vi "LibraryTest.vi"() -> ()   [LabVIEW 2019]
uses:
  <vilib>/ptbypt/NI_PtbyPt.lvlib
panel:
  in  "ipAddress 2":string="192.168.254.1"
  out "Sample dt (ms)":dbl format="%0.2f"
  in  "stop":bool
  out "length":i32
  out "error out":errorcluster
  out "return 2":string
  out "qtmPort":i32
  out "ipAddress":string
  out "return":i32
  # "IP Address of the PC running QTM"
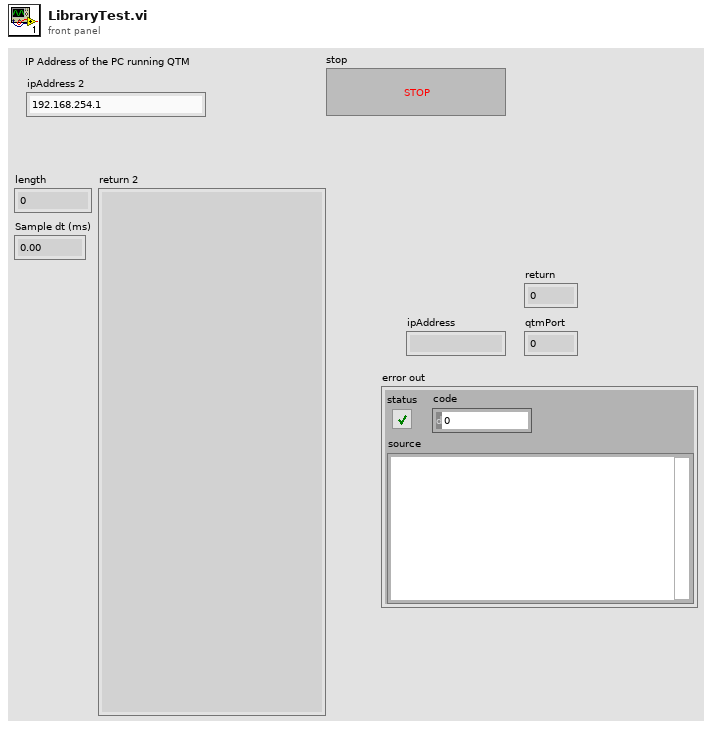
[diagram p1: front panel]
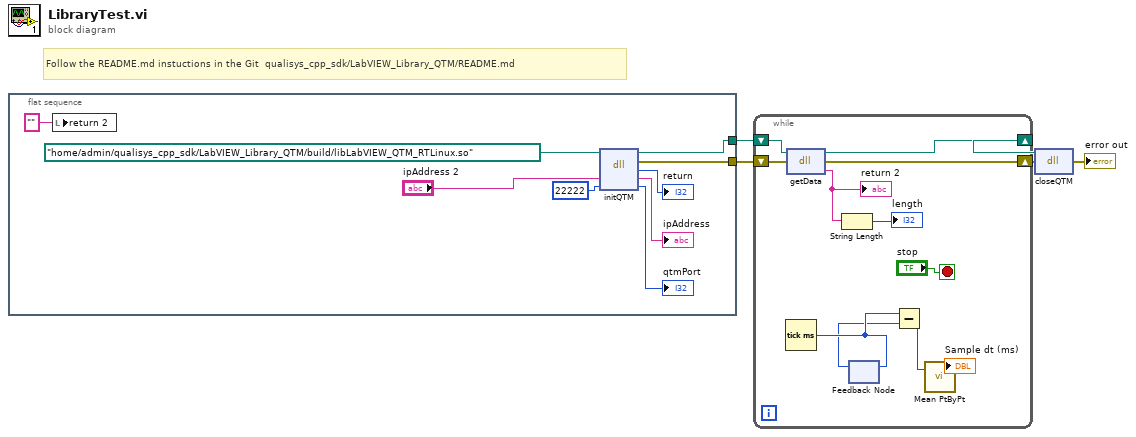
[diagram p0: block diagram]
diagram:
  # "Follow the README.md instuctions in the Git  qualisys_cpp_sdk/LabVIEW_Library_QTM/README.md"
  n1 = flat-sequence {
    tunnel: [w8] -> w5
    tunnel: [w7] -> w3
    frame #0 {
      n2 = local write "return 2"("") -> ()
      n3 = dll-call lib="home/admin/qualisys_cpp_sdk/LabVIEW_Library_QTM/build/libLabVIEW_QTM_RTLinux.so" fn="initQTM"(path in=path "/home/admin/qualisys_cpp_sdk/LabVIEW_Library_QTM/build/libLabVIEW_QTM_RTLinux.so", "ipAddress"="ipAddress 2", "qtmPort"=22222) -> (path out=w8:path, error out=w7:errorcluster, "return"=→"return":i32, "ipAddress"=→"ipAddress":string, "qtmPort"=→"qtmPort":i32)  [unwired: 2 in]
    }
  }
  n4 = while {
    shift-right: [w24] -> w4
    shift-left: w5 -> [w25]
    shift-right: [w22] -> w2
    shift-left: w3 -> [w23]
    stop <- "stop" stop-if-true
    n5 = Tick Count (ms)() -> (millisecond timer value=w18:u32)
    n6 = dll-call lib="home/admin/qualisys_cpp_sdk/LabVIEW_Library_QTM/build/libLabVIEW_QTM_RTLinux.so" fn="getData"(path in=w25, error in=w23) -> (path out=w24:path, error out=w22:errorcluster, "return"=w20:string)  [unwired: 1 in]
    "return 2" <- w20
    n7 = String Length(string=w20) -> (length=→"length":i32)
    n8 = feedback-in #1(w18) -> ()
    n9 = feedback #1() -> (w17:u32)  [unwired: 1 in]
    n10 = Subtract(x=w18, y=w17) -> (x-y=w16:u32)
    n11 = call <vilib>:"Mean PtByPt.vi"("x"=w16) -> ("mean"=→"Sample dt (ms)":dbl)  [unwired: 3 in, 1 out]
  }
  n12 = dll-call lib="home/admin/qualisys_cpp_sdk/LabVIEW_Library_QTM/build/libLabVIEW_QTM_RTLinux.so" fn="closeQTM"(path in=w4, error in=w2) -> (error out=→"error out":errorcluster)  [unwired: 2 in, 1 out]
